vi "Create.vi"(8 "error in (no error)":errorcluster) -> (0 "error out":errorcluster, 2 "TimerAPI":refnum<class "TimerAPI.lvclass">, 3 "Timing Module out":refnum<class "Timing Module.lvclass">)   [LabVIEW 2020, in "Volatus.lvlib" / "Timing Module.lvclass"]
uses:
  Timing Module.lvclass
  Timing Module.lvclass/Timing Module.ctl
  TimerAPI/TimerAPI.lvclass
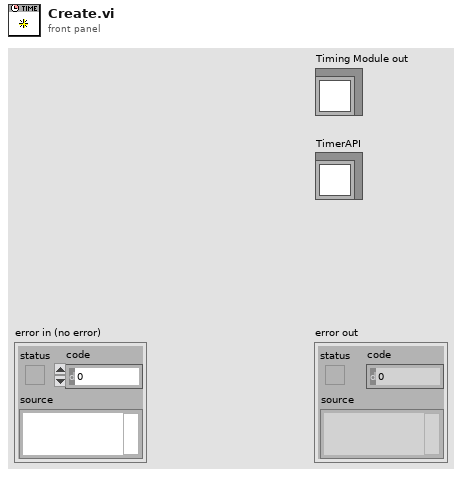
[diagram p1: front panel]
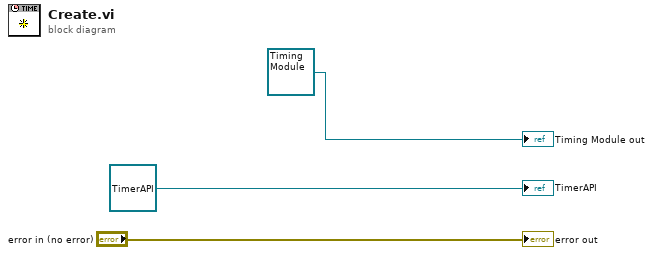
[diagram p0: block diagram]
diagram:
  "error out" <- "error in (no error)"
  "Timing Module out" <- refnum<class "Timing Module.lvclass"> refnum ("Timing Module in")
  "TimerAPI" <- refnum<class "TimerAPI.lvclass"> refnum ("Volatus:TimerAPI.lvclass")
